vi "功能走合判定.vi"(0 "曲线引用":refnum<vi>, 1 "功能":T1, 3 "错误输入":errorcluster) -> (7 "曲线引用输出":refnum<vi>, 8 "OK":bool, 10 "错误输出":errorcluster)   [LabVIEW 2018]
uses:
  <userlib>/_MGI/1D Array/MGI Average/MGI Average (DBL[]).vi
  Global_Variable/Global.vi
  Global_Variable/A180648.vi
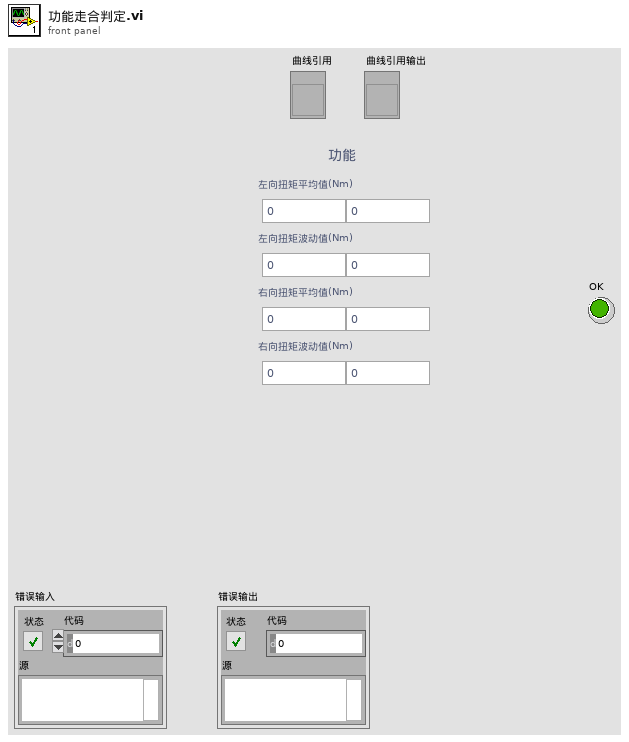
[diagram p1: front panel]
types:
  T1 = cluster{"左向扭矩平均值(Nm)":cluster{"下限":dbl, "上限":dbl}, "左向扭矩波动值(Nm)":cluster{"下限":dbl, "上限":dbl}, "右向扭矩平均值(Nm)":cluster{"下限":dbl, "上限":dbl}, "右向扭矩波动值(Nm)":cluster{"下限":dbl, "上限":dbl}}
  T2 = enum32{"空载", "功能", "力特性", "传感器特性", "电流特性", "振动NVH", "逆向空载", "完成"}
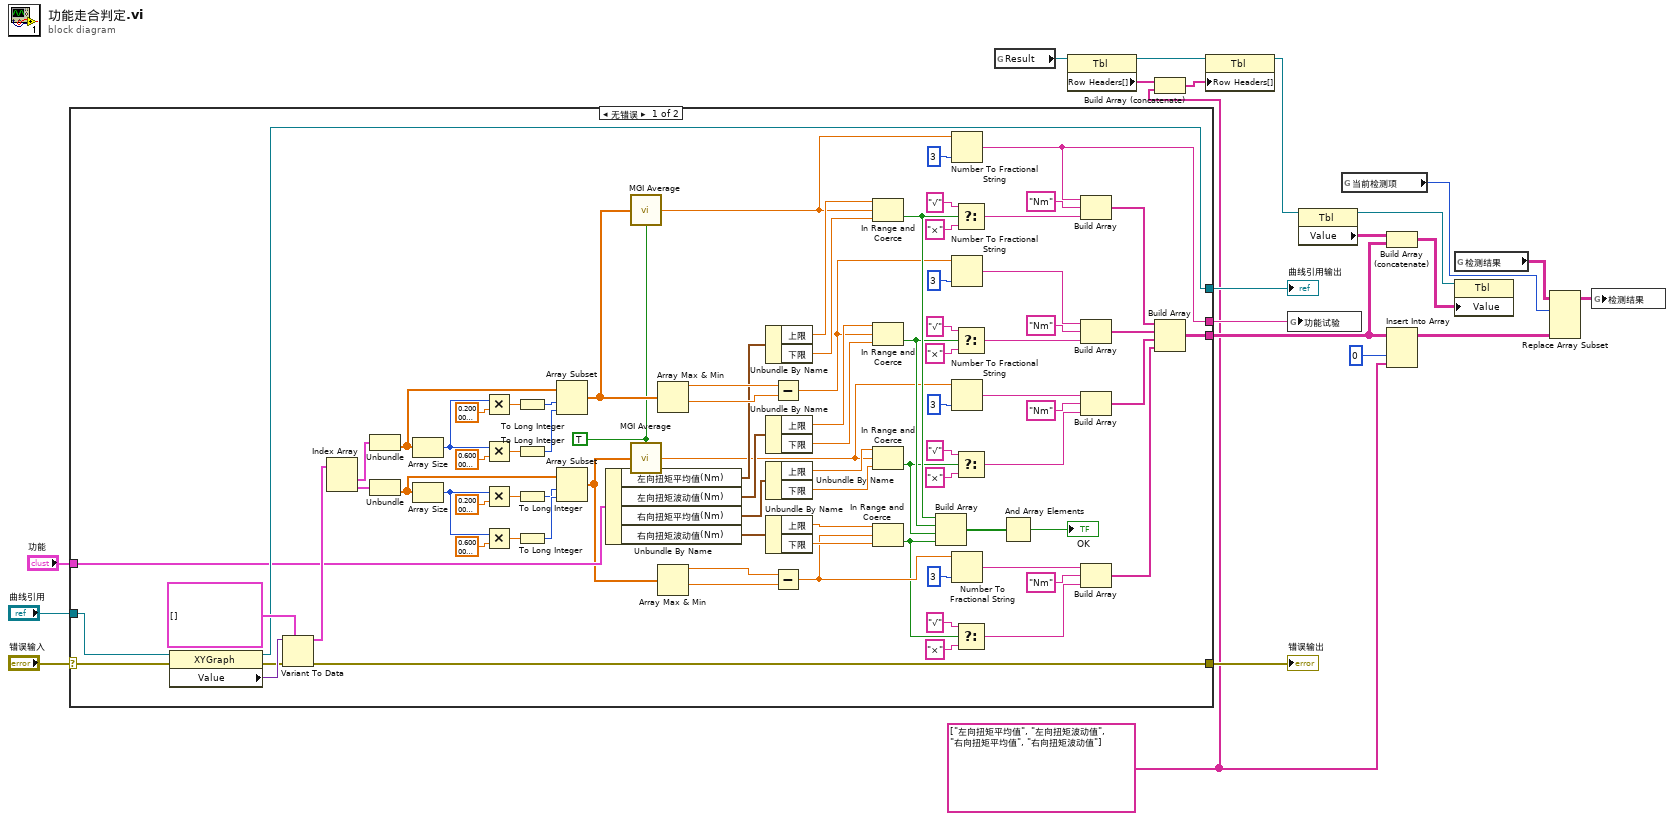
[diagram p0: block diagram]
diagram:
  w3 = string[] ["左向扭矩平均值", "左向扭矩波动值", "右向扭矩平均值", "右向扭矩波动值"] ("元素")
  n1 = case shown="无错误" "错误输入" {
    selector: "错误输入" -> [w104 w108]
    tunnel: [w100 w108] -> w20
    tunnel: "曲线引用" -> [w103 w107]
    tunnel: [w102 w107] -> w18
    tunnel: "功能" -> [w82 _]
    tunnel: [w63 _] -> w4
    tunnel: [w26 _] -> w8
    frame No Error {
      w55 = TRUE ("Ignore NaN? (F)")
      n2 = property class="XYGraph"(reference=w103, error in=w104) -> (reference out=w102:refnum<vi>, error out=w101:errorcluster, "Value"=w106:variant)
      n3 = Variant To Data(error in=w101, type=cluster{dbl[], dbl[]}[] [], Variant=w106) -> (data=w92:cluster{dbl[], dbl[]}[], error out=w100:errorcluster)
      n4 = Index Array(array=w92) -> (element #1=w91:cluster{dbl[], dbl[]}, element #2=w83:cluster{dbl[], dbl[]})  [unwired: 2 in]
      n5 = Unbundle(w91) -> (w81:dbl[])  [unwired: 1 out]
      n6 = Unbundle(w83) -> (w80:dbl[])  [unwired: 1 out]
      n7 = Array Size(array=w81) -> (size(s)=w93:i32)
      n8 = Array Size(array=w80) -> (size(s)=w90:i32)
      n9 = Multiply(x=w93, y=sgl 0.2) -> (x*y=w97:sgl)
      n10 = Multiply(x=w93, y=sgl 0.6) -> (x*y=w98:sgl)
      n11 = Multiply(x=w90, y=sgl 0.2) -> (x*y=w86:sgl)
      n12 = Multiply(x=w90, y=sgl 0.6) -> (x*y=w85:sgl)
      n13 = To Long Integer(number=w97) -> (32bit integer=w99:i32)
      n14 = To Long Integer(number=w98) -> (32bit integer=w94:i32)
      n15 = To Long Integer(number=w86) -> (32bit integer=w84:i32)
      n16 = To Long Integer(number=w85) -> (32bit integer=w89:i32)
      n17 = Array Subset(array=w81, index=w99, length=w94) -> (w61:dbl[])
      n18 = Array Subset(array=w80, index=w84, length=w89) -> (w62:dbl[])
      n19 = Unbundle By Name(w82) -> ("左向扭矩平均值(Nm)"=w39:cluster{"下限":dbl, "上限":dbl}, "左向扭矩波动值(Nm)"=w38:cluster{"下限":dbl, "上限":dbl}, "右向扭矩平均值(Nm)"=w31:cluster{"下限":dbl, "上限":dbl}, "右向扭矩波动值(Nm)"=w30:cluster{"下限":dbl, "上限":dbl})
      n20 = call-poly <userlib>:"MGI Average.vi"("Double[]"=w61, "Ignore NaN? (F)"=w55) -> ("Average"=w37:dbl)
      n21 = call-poly <userlib>:"MGI Average.vi"("Double[]"=w62, "Ignore NaN? (F)"=w55) -> ("Average"=w28:dbl)
      n22 = Array Max & Min(array=w61) -> (max value=w60:dbl, min value=w59:dbl)  [unwired: 2 out]
      n23 = Array Max & Min(array=w62) -> (max value=w58:dbl, min value=w57:dbl)  [unwired: 2 out]
      n24 = Unbundle By Name(w39) -> ("上限"=w43:dbl, "下限"=w42:dbl)
      n25 = Unbundle By Name(w38) -> ("上限"=w41:dbl, "下限"=w40:dbl)
      n26 = Unbundle By Name(w31) -> ("上限"=w79:dbl, "下限"=w78:dbl)
      n27 = Unbundle By Name(w30) -> ("上限"=w56:dbl, "下限"=w29:dbl)
      n28 = Subtract(x=w60, y=w59) -> (x-y=w34:dbl)
      n29 = Subtract(x=w58, y=w57) -> (x-y=w27:dbl)
      n30 = In Range and Coerce(upper limit=w43, x=w37, lower limit=w42) -> (In Range?=w35:bool)  [unwired: 1 out]
      n31 = In Range and Coerce(upper limit=w41, x=w34, lower limit=w40) -> (In Range?=w32:bool)  [unwired: 1 out]
      n32 = In Range and Coerce(upper limit=w79, x=w28, lower limit=w78) -> (In Range?=w25:bool)  [unwired: 1 out]
      n33 = In Range and Coerce(upper limit=w56, x=w27, lower limit=w29) -> (In Range?=w24:bool)  [unwired: 1 out]
      n34 = Build Array(w35, w32, w25, w24) -> (w65:bool[])
      n35 = Number To Fractional String(number=w37, precision (6)=i16 3 ("精度(6)")) -> (F-format string=w26:string)  [unwired: 2 in]
      n36 = Number To Fractional String(number=w34, precision (6)=i16 3 ("精度(6)")) -> (F-format string=w54:string)  [unwired: 2 in]
      n37 = Number To Fractional String(number=w28, precision (6)=i16 3 ("精度(6)")) -> (F-format string=w76:string)  [unwired: 2 in]
      n38 = Number To Fractional String(number=w27, precision (6)=i16 3 ("精度(6)")) -> (F-format string=w67:string)  [unwired: 2 in]
      n39 = Select(t="√", s=w35, f="×") -> (s? t:f=w44:string)
      n40 = Select(t="√", s=w32, f="×") -> (s? t:f=w53:string)
      n41 = Select(t="√", s=w25, f="×") -> (s? t:f=w72:string)
      n42 = Select(t="√", s=w24, f="×") -> (s? t:f=w71:string)
      n43 = And Array Elements(Boolean array=w65) -> (logical AND=→"OK":bool)
      n44 = Build Array(w26, "Nm" ("元素"), w44) -> (w36:string[])
      n45 = Build Array(w54, "Nm" ("元素"), w53) -> (w33:string[])
      n46 = Build Array(w76, "Nm" ("元素"), w72) -> (w23:string[])
      n47 = Build Array(w67, "Nm" ("元素"), w71) -> (w22:string[])
      n48 = Build Array(w36, w33, w23, w22) -> (w63:string[][])
    }
    frame Error {
    }
  }
  "错误输出" <- w20
  "曲线引用输出" <- w18
  n49 = global read "Global.vi" "Result"() -> (w17:refnum<vi>)
  n50 = property class="Tbl"(reference=w17) -> (reference out=w14:refnum<vi>, "Row Headers[]"=w16:string[])  [unwired: 1 in, 1 out]
  n51 = Build Array (concatenate)(w16, w3) -> (w15:string[])
  n52 = property class="Tbl"(reference=w14, "Row Headers[]"=w15) -> (reference out=w13:refnum<vi>)  [unwired: 1 in, 1 out]
  n53 = global write "检测结果.vi" "功能试验"(w8) -> ()
  n54 = property class="Tbl"(reference=w13) -> (reference out=w12:refnum<vi>, "Value"=w11:string[][])  [unwired: 1 in, 1 out]
  n55 = global read "A180648.vi" "当前检测项"() -> (w6:T2)
  n56 = Build Array (concatenate)(w11, w4) -> (w10:string[][])
  n57 = Insert Into Array(array=w4, index (col)=0 ("禁用的索引 (列)"), new element=w3) -> (w1:string[][])  [unwired: 1 in]
  n58 = global read "A180648.vi" "检测结果"() -> (w7:string[][][])
  n59 = property class="Tbl"(reference=w12, "Value"=w10) -> ()  [unwired: 1 in, 2 out]
  n60 = Replace Array Subset(array=w7, new element=w1, index (dim 0)=w6) -> (w5:string[][][])  [unwired: 2 in]
  n61 = global write "A180648.vi" "检测结果"(w5) -> ()
